vi "Write-Data.vi"(8 "error in (no error)":errorcluster, 10 "Data":dbl[](array[numeric]), 11 "Modbus-Instr in":refnum<class "Modbus-Instr.lvclass">) -> (0 "error out":errorcluster, 3 "Modbus-Instr out":refnum<class "Modbus-Instr.lvclass">)   [LabVIEW 2021, in "Modbus-Instr.lvclass"]
uses:
  Modbus-Instr.lvclass
  Modbus-Instr.lvclass/Modbus-Instr.ctl
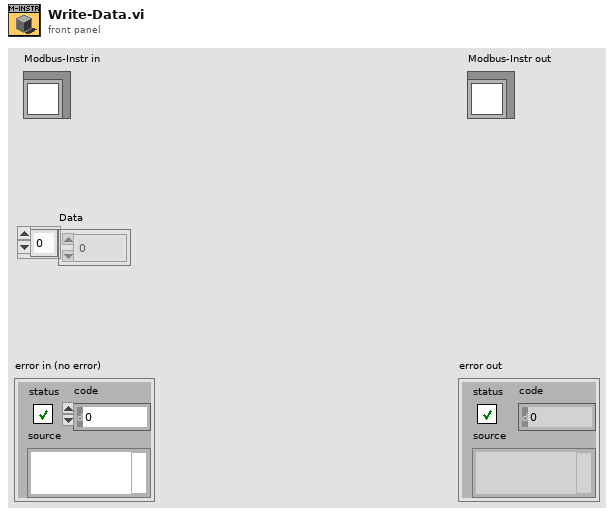
[diagram p1: front panel]
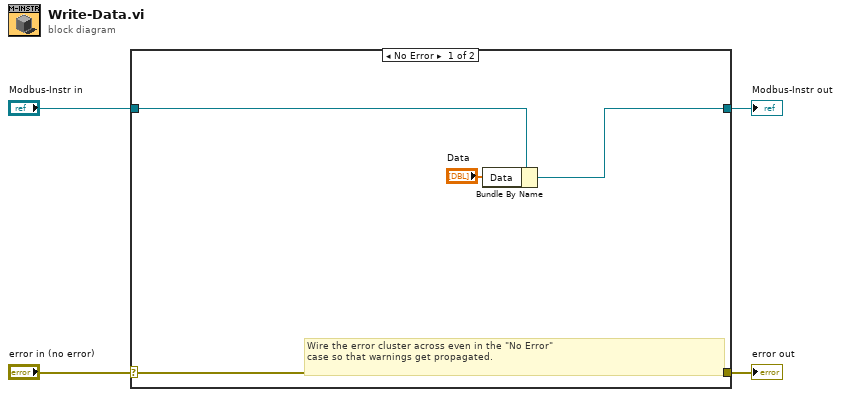
[diagram p0: block diagram]
diagram:
  n1 = case shown="No Error" "error in (no error)" {
    selector: "error in (no error)" -> [w8 w10]
    tunnel: [w8 w10] -> w3
    tunnel: [w6 w9] -> w1
    tunnel: "Modbus-Instr in" -> [w7 w9]
    frame No Error {
      # "Wire the error cluster across even in the \"No Error\"\ncase so that warnings get propagated."
      n2 = Bundle By Name(cluster=w7, "Data"="Data") -> (w6:refnum<class "Modbus-Instr.lvclass">)
    }
    frame Error {
    }
  }
  "error out" <- w3
  "Modbus-Instr out" <- w1
